vi "SLSC Get Plugin Path.vi"(9 "Type":string="_pinout.png", 10 "number":i32, 11 "Vendor Prefix":string) -> (3 "appended path":path)   [LabVIEW 2024, in "SLSC EDS System Explorer.lvlib"]
uses:
  SLSC EDS System Explorer.lvlib
  C:/Users/ppathak/Downloads/NationalInstruments.VeriStand.dll
  Users/ppathak/Downloads/NationalInstruments.VeriStand.dll
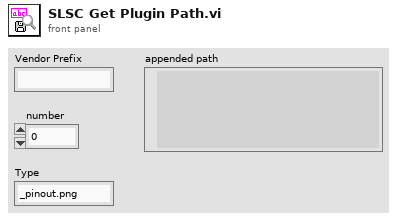
[diagram p1: front panel]
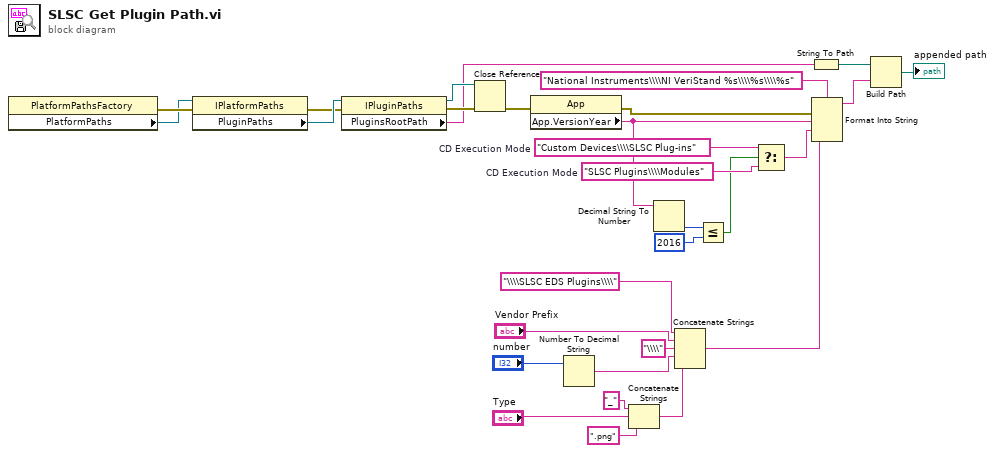
[diagram p0: block diagram]
diagram:
  w22 = "SLSC Plugins\\\\Modules"  # CD Execution Mode
  w23 = "Custom Devices\\\\SLSC Plug-ins"  # CD Execution Mode
  n1 = property class="PlatformPathsFactory"() -> (error out=w7:errorcluster, "PlatformPaths"=w5:refnum<k24>)  [unwired: 2 in, 1 out]
  n2 = property class="IPlatformPaths"(reference=w5, error in=w7) -> (error out=w6:errorcluster, "PluginPaths"=w8:refnum<k24>)  [unwired: 1 out]
  n3 = property class="IPluginPaths"(reference=w8, error in=w6) -> (reference out=w3:refnum<k24>, error out=w4:errorcluster, "PluginsRootPath"=w2:string)
  n4 = Close Reference(reference=w3, error in (no error)=w4) -> (error out=w1:errorcluster)
  n5 = property class="App"(error in=w1) -> (error out=w15:errorcluster, "App.VersionYear"=w17:string)  [unwired: 1 in, 1 out]
  n6 = Number To Decimal String(number="number") -> (decimal integer string=w26:string)  [unwired: 1 in]
  n7 = Concatenate Strings("_" ("string"), "Type", ".png" ("string")) -> (w10:string)
  n8 = Decimal String To Number(string=w17) -> (number=w18:i32)  [unwired: 2 in, 1 out]
  n9 = Concatenate Strings("\\\\SLSC EDS Plugins\\\\" ("string"), "Vendor Prefix", "\\\\" ("string"), w26, w10) -> (w27:string)
  n10 = Less Or Equal?(x=w18, y=2016) -> (x <= y?=w21:bool)
  n11 = Select(t=w23, s=w21, f=w22) -> (s? t:f=w20:string)
  n12 = String To Path(string=w2) -> (path=w9:path)
  n13 = Format Into String(format string="National Instruments\\\\NI VeriStand %s\\\\%s\\\\%s" ("name or relative path"), error in=w15, w17, w20, w27) -> (resulting string=w14:string)  [unwired: 1 in, 1 out]
  n14 = Build Path(base path=w9, name or relative path=w14) -> (appended path=→"appended path":path)
